vi "TxP Configure.vi"(0 "Instrument Handle In":refnum<k21>, 1 "Selector String":string, 5 "TxP Config":T1={"Measurement Interval (s)"=0.001, "RBW"={"RBW Filter Type"=1, "RBW (Hz)"=100000.0, "RRC Alpha"=0.01}, "VBW"={"VBW Auto"=1, "VBW (Hz)"=30000.0, "VBW to RBW Ratio"=3.0}, "Threshold"={"Threshold Enabled"=0, "Threshold Type"=0, "Threshold Level (dB or dBm)"=-20.0}, "Averaging"={"Averaging Count"=10, "Averaging Enabled"=0, "Averaging Type"=0}} {"Averaging"."Averaging Type" items=["RMS", "Log", "Scalar", "Max", "Min"]; "Averaging"."Averaging Enabled" items=["False", "True"]; "Threshold"."Threshold Level (dB or dBm)" format="%.2g"; "Threshold"."Threshold Type" items=["Relative", "Absolute"]; "Threshold"."Threshold Enabled" items=["False", "True"]; "VBW"."VBW to RBW Ratio" format="%#.6f"; "VBW"."VBW (Hz)" format="%.3p"; "VBW"."VBW Auto" items=["False", "True"]; "RBW"."RRC Alpha" format="%.3g"; "RBW"."RBW (Hz)" format="%.3p"; "RBW"."RBW Filter Type" items=["None"=5, "Gaussian"=1, "Flat"=2, "RRC"=6]; "Measurement Interval (s)" format="%.2p"}, 11 "error in (no error)":errorcluster) -> (4 "Instrument Handle Out":refnum<k21>, 15 "error out":errorcluster)   [LabVIEW 2016, in "RFmxSpecAn.lvlib"]
uses:
  RFmxSpecAn.lvlib
  <resource>/objmgr/RFmxSpecAn.rc
  Typedefs/TxP Configuration.ctl
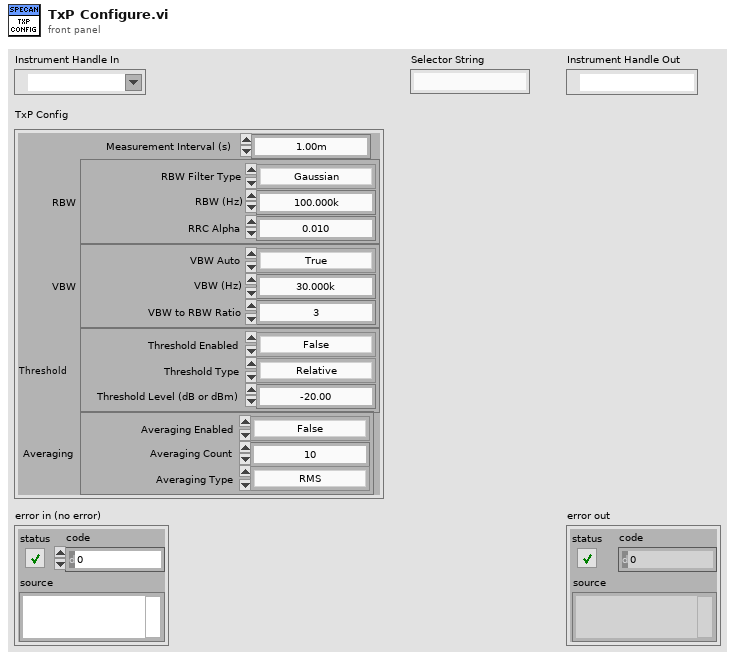
[diagram p1: front panel]
types:
  T1 = typedef "RFmxSpecAn.lvlib/TxP Configuration.ctl" = cluster{"Measurement Interval (s)":dbl, "RBW":cluster{"RBW Filter Type":i32, "RBW (Hz)":dbl, "RRC Alpha":dbl}, "VBW":cluster{"VBW Auto":i32, "VBW (Hz)":dbl, "VBW to RBW Ratio":dbl}, "Threshold":cluster{"Threshold Enabled":i32, "Threshold Type":i32, "Threshold Level (dB or dBm)":dbl}, "Averaging":cluster{"Averaging Count":i32, "Averaging Enabled":i32, "Averaging Type":i32}}
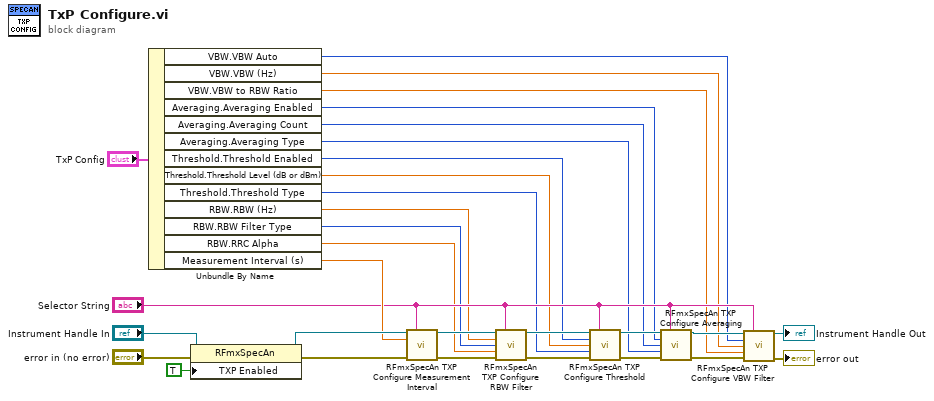
[diagram p0: block diagram]
diagram:
  n1 = Unbundle By Name("TxP Config") -> ("VBW.VBW Auto"=w1:i32, "VBW.VBW (Hz)"=w2:dbl, "VBW.VBW to RBW Ratio"=w3:dbl, "Averaging.Averaging Enabled"=w4:i32, "Averaging.Averaging Count"=w5:i32, "Averaging.Averaging Type"=w6:i32, "Threshold.Threshold Enabled"=w7:i32, "Threshold.Threshold Level (dB or dBm)"=w8:dbl, "Threshold.Threshold Type"=w9:i32, "RBW.RBW (Hz)"=w10:dbl, "RBW.RBW Filter Type"=w11:i32, "RBW.RRC Alpha"=w12:dbl, "Measurement Interval (s)"=w14:dbl)
  n2 = property class="RFmxSpecAn"(reference="Instrument Handle In", error in="error in (no error)", "TXP Enabled"=TRUE) -> (reference out=w19:refnum<k21>, error out=w30:errorcluster)
  n3 = call <vilib>:"RFmxSpecAn TXP Configure Measurement Interval.vi"("Instrument Handle In"=w19, "Selector String"="Selector String", "Measurement Interval (s)"=w14, "error in (no error)"=w30) -> ("Instrument Handle Out"=w29:refnum<k21>, "error out"=w28:errorcluster)  [unwired: 10 in]
  n4 = call <vilib>:"RFmxSpecAn TXP Configure RBW Filter.vi"("Instrument Handle In"=w29, "Selector String"="Selector String", "RBW (Hz)"=w10, "RBW Filter Type"=w11, "RRC Alpha"=w12, "error in (no error)"=w28) -> ("Instrument Handle Out"=w26:refnum<k21>, "error out"=w27:errorcluster)  [unwired: 8 in]
  n5 = call <vilib>:"RFmxSpecAn TXP Configure Threshold.vi"("Instrument Handle In"=w26, "Selector String"="Selector String", "Threshold Enabled"=w7, "Threshold Level (dB or dBm)"=w8, "Threshold Type"=w9, "error in (no error)"=w27) -> ("Instrument Handle Out"=w25:refnum<k21>, "error out"=w24:errorcluster)  [unwired: 8 in]
  n6 = call <vilib>:"RFmxSpecAn TXP Configure Averaging.vi"("Instrument Handle In"=w25, "Selector String"="Selector String", "Averaging Enabled"=w4, "Averaging Count"=w5, "Averaging Type"=w6, "error in (no error)"=w24) -> ("Instrument Handle Out"=w23:refnum<k21>, "error out"=w22:errorcluster)  [unwired: 8 in]
  n7 = call <vilib>:"RFmxSpecAn TXP Configure VBW Filter.vi"("Instrument Handle In"=w23, "Selector String"="Selector String", "VBW Auto"=w1, "VBW (Hz)"=w2, "VBW to RBW Ratio"=w3, "error in (no error)"=w22) -> ("Instrument Handle Out"=→"Instrument Handle Out":refnum<k21>, "error out"=→"error out":errorcluster)  [unwired: 8 in]
